vi "GetMsgData.vi"(8 "error in (no error)":errorcluster, 11 "PrintF in":refnum<class "PrintF.lvclass">) -> (0 "error out":errorcluster, 2 "MsgData":variant, 3 "PrintF out":refnum<class "PrintF.lvclass">)   [LabVIEW 2020, in "UpstreamMsg.lvlib" / "PrintF.lvclass"]
doc: "This is used in the scripting to create the go, it provides the datatype"
uses:
  PrintF.lvclass
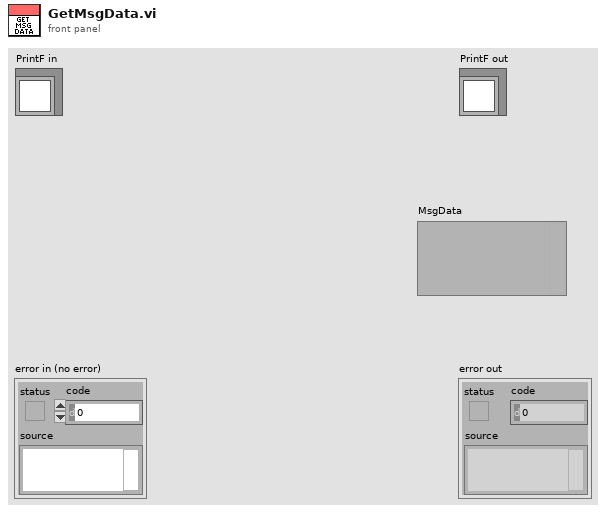
[diagram p1: front panel]
types:
  T1 = typedef "UpstreamMsg.lvlib/PrintF.lvclass/Msg.ctl" = cluster{"TxtColor":cluster{"r":u8, "b":u8, "g":u8}, "LineToPrint":string}
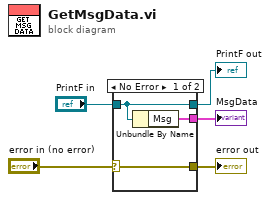
[diagram p0: block diagram]
diagram:
  n1 = case shown="No Error" "error in (no error)" {
    selector: "error in (no error)" -> [w8 w10]
    tunnel: [w8 w10] -> w5
    tunnel: [w7 w9] -> w3
    tunnel: "PrintF in" -> [w7 w9]
    tunnel: [w6 _] -> w4
    frame No Error {
      n2 = Unbundle By Name(w7) -> ("Msg"=w6:T1)
    }
    frame Error {
    }
  }
  "error out" <- w5
  "PrintF out" <- w3
  "MsgData" <- w4
